vi "EditOptions.vi"(8 "error in":errorcluster, 11 "node in":refnum<class "RunTimeMenuItem.lvclass">) -> (0 "error out":errorcluster, 1 "edit options":T1, 2 "subnodes class":T2, 3 "node out":refnum<class "RunTimeMenuItem.lvclass">)   [LabVIEW 2019, in "RunTimeMenuItem.lvclass"]
doc: "Contains the options for the Menu that will be displayed when doing right click on an item.\nThe sub nodes class configures which nodes can be added to this nodes\nAnd the edit options determine which options are available for the node.\nThis configuration is stored in this VI in case some dynamic configuration is required for the menu options or sub nodes."
uses:
  RunTimeMenuItem.lvclass
  <vilib>/NI/Configuration Framework/Node/SubNodeCluster.ctl
  <vilib>/NI/Configuration Framework/Node/NodeMenuOptions.ctl
  <vilib>/NI/Configuration Framework/Node/NISE_CEF_Node.lvclass
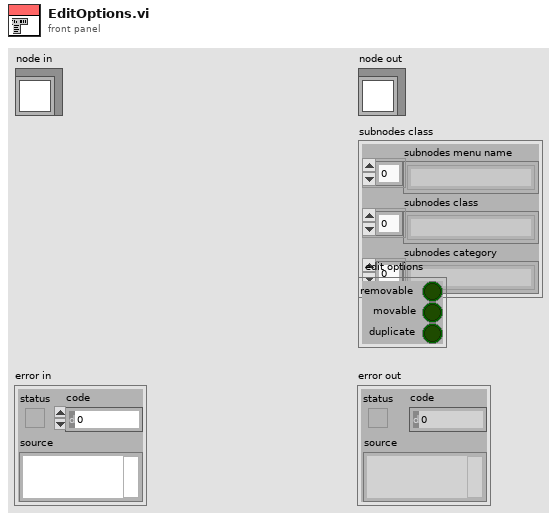
[diagram p1: front panel]
types:
  T1 = typedef "NISE_CEF_Node.lvclass/NodeMenuOptions.ctl" = cluster{"removable":bool, "movable":bool, "duplicate":bool}
  T2 = typedef "NISE_CEF_Node.lvclass/SubNodeCluster.ctl" = cluster{"subnodes menu name":string[], "subnodes class":string[], "subnodes category":string[]}
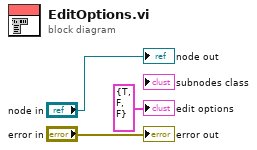
[diagram p0: block diagram]
diagram:
  "error out" <- "error in"
  "node out" <- "node in"
  "edit options" <- T1 {"removable"=TRUE, "movable"=FALSE, "duplicate"=FALSE} ("edit options")
